vi "ma_sml_Compute H(w) from h(n).vi"(0 "h":dbl[](array[numeric]) format="%.2f", 1 "FFT size":i32=1024) -> (2 "Mag H(w)":dbl[](array[numeric]) format="%.2f", 3 "Phase H(w)":dbl[](array[numeric]) format="%.2f", 4 "df":dbl format="%.2f")   [LabVIEW 2020, in "NI_MAPro.lvlib"]
uses:
  NI_MAPro.lvlib
  NI_AALPro.lvlib
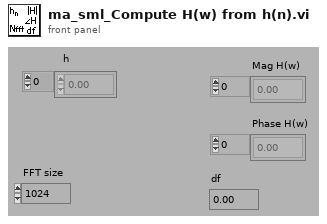
[diagram p1: front panel]
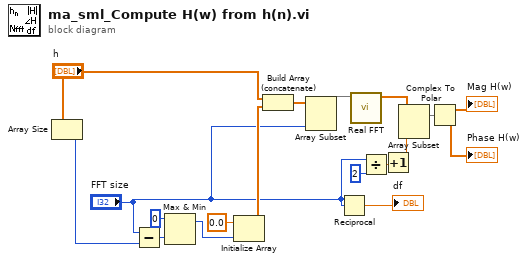
[diagram p0: block diagram]
diagram:
  n1 = Array Size(array="h") -> (size(s)=w12:i32)
  n2 = Subtract(x="FFT size", y=w12) -> (x-y=w6:i32)
  n3 = Max & Min(x=0, y=w6) -> (max(x,y)=w4:i32)  [unwired: 1 out]
  n4 = Initialize Array(0.0, w4) -> (w11:dbl[])
  n5 = Build Array (concatenate)("h", w11) -> (w3:dbl[])
  n6 = Array Subset(array=w3, length="FFT size") -> (w2:dbl[])  [unwired: 1 in]
  n7 = Reciprocal(x="FFT size") -> (1/x=→"df":dbl)
  n8 = call "Real FFT.vi"("X"=w2) -> ("FFT {X}"=w10:cdb[])  [unwired: 9 in, 1 out]
  n9 = Divide(x="FFT size", y=2) -> (x/y=w17:dbl)
  n10 = Increment(x=w17) -> (x+1=w16:dbl)
  n11 = Array Subset(array=w10, length=w16) -> (w9:cdb[])  [unwired: 1 in]
  n12 = Complex To Polar(r * e^(i*theta)=w9) -> (r=→"Mag H(w)":dbl[], theta=→"Phase H(w)":dbl[])
